vi "Console.vi"(0 "Translate":enum16{"None", "Tiny", "URAPI"}(ring), 3 "Reply":string, 4 "Variables":u16[](array[numeric]), 5 "Sent":string[](array[string])) -> (1 "Variables":string, 2 "BotSpeak":string)   [LabVIEW 2014]
panel:
  out "Console":string
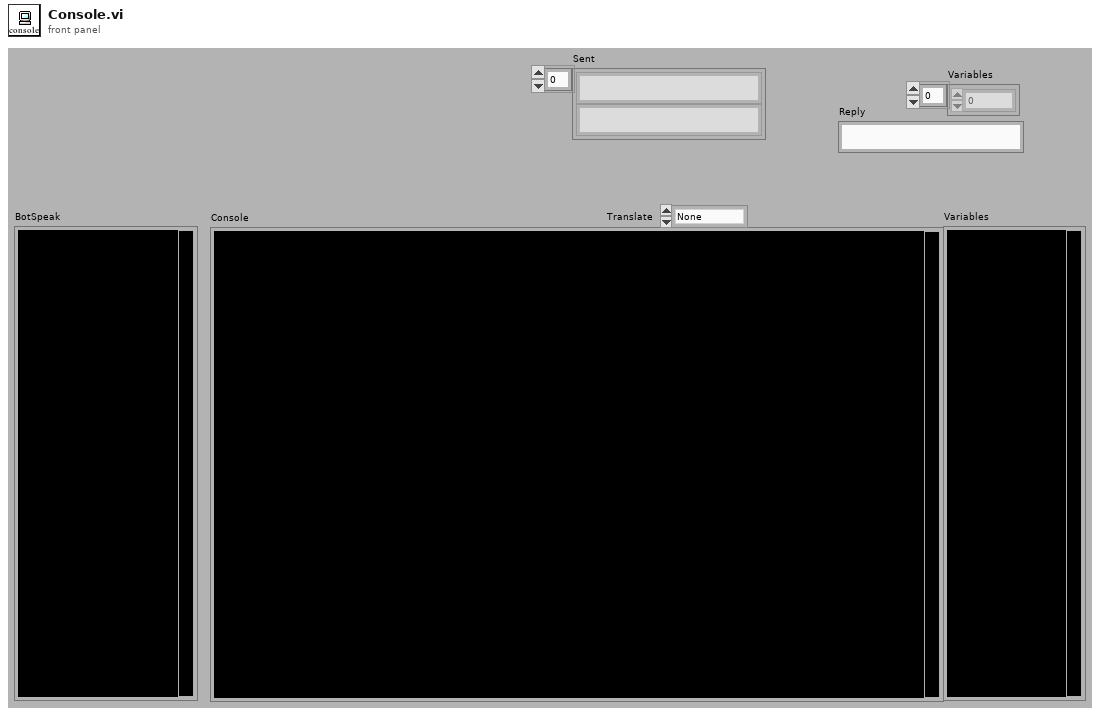
[diagram p1: front panel]
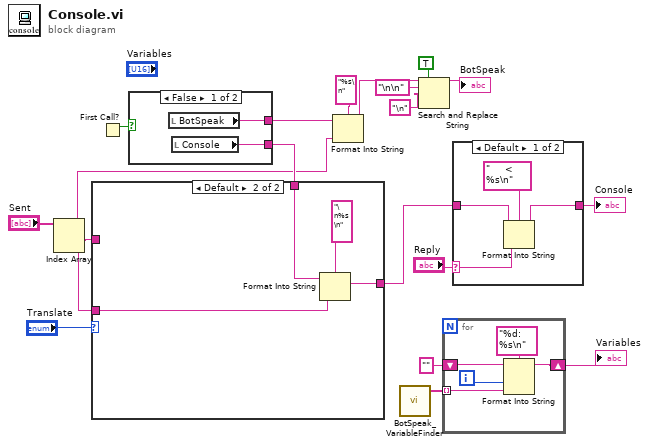
[diagram p0: block diagram]
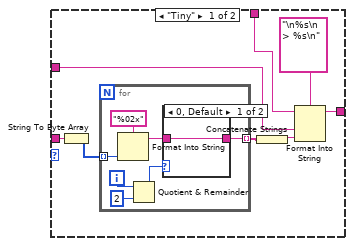
[diagram p2: hidden frame]
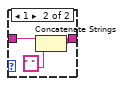
[diagram p3: hidden frame]
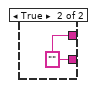
[diagram p5: hidden frame]
diagram:
  n1 = Index Array(array="Sent") -> (element #1=w8:string, element #2=w18:string)  [unwired: 2 in]
  n2 = First Call?() -> (First Call?: T/F=w14:bool)
  n3 = case shown="False" w14 {
    tunnel: [w21 w22] -> w10
    tunnel: [w20 w22] -> w7
    frame False {
      n4 = local read "BotSpeak"() -> (w20:string)
      n5 = local read "Console"() -> (w21:string)
    }
    frame True {
      w22 = "" ("Console")
    }
  }
  n6 = case shown="Default" "Translate" {
    tunnel: w18 -> [w30 w43]
    tunnel: w8 -> [w25 _]
    tunnel: w10 -> [w24 w44]
    tunnel: [w23 w42] -> w9
    frame "Tiny" {
      n7 = String To Byte Array(string=w30) -> (unsigned byte array=w29:u8[])
      n8 = for {
        tunnel: w29 -> [w37] mode=indexing
        tunnel: [w31] -> w28 mode=indexing
        i -> [w35]
        n9 = Format Into String(format string="%02x", w37) -> (resulting string=w32:string)  [unwired: 2 in, 1 out]
        n10 = Quotient & Remainder(x=w35, y=2) -> (x-y*floor(x/y)=w33:i32)  [unwired: 1 out]
        n11 = case shown="0, Default" w33 {
          tunnel: w32 -> [w38 w41]
          tunnel: [w38 w39] -> w31
          frame 0, Default {
          }
          frame 1 {
            n12 = Concatenate Strings(w41, " " ("format string")) -> (w39:string)
          }
        }
      }
      n13 = Concatenate Strings(w28) -> (w26:string)
      n14 = Format Into String(format string="\n%s\n     > %s\n", initial string=w24, w25, w26) -> (resulting string=w23:string)  [unwired: 1 in, 1 out]
    }
    frame Default {
      n15 = Format Into String(format string="\n%s\n", initial string=w44, w43) -> (resulting string=w42:string)  [unwired: 1 in, 1 out]
    }
  }
  n16 = Format Into String(format string="%s\n", initial string=w7, w8) -> (resulting string=w5:string)  [unwired: 1 in, 1 out]
  n17 = call <userlib>:"BotSpeak_VariableFinder.vi"() -> ("Variables"=w17:string[])  [unwired: 3 in, 1 out]
  n18 = Search and Replace String(replace all?=TRUE ("replace all? (F)"), input string=w5, search string="\n\n", replace string="\n" ("search string")) -> (result string=→"BotSpeak":string)  [unwired: 4 in, 3 out]
  n19 = for {
    tunnel: w17 -> [w48] mode=indexing
    shift-right: [w47] -> w15
    shift-left: "" -> [w46]
    i -> [w49]
    n20 = Format Into String(format string="%d: %s\n", initial string=w46, w49, w48) -> (resulting string=w47:string)  [unwired: 1 in, 1 out]
  }
  "Variables" <- w15
  n21 = case shown="Default" "Reply" {
    selector: "Reply" -> [w53 _]
    tunnel: [w51 w55] -> w12
    tunnel: w9 -> [w52 w55]
    frame Default {
      n22 = Format Into String(format string="     < %s\n", initial string=w52, w53) -> (resulting string=w51:string)  [unwired: 1 in, 1 out]
    }
    frame "" {
    }
  }
  "Console" <- w12
